vi "LIN UDS Response.vi"(6 "TimeOutMs":i32, 7 "pResData":u8[](array[numeric])=array[4097 elements], 8 "error in (no error)":errorcluster, 9 "pUDSAddr":T1, 10 "LINIndex":u8, 11 "DevHandle":i32) -> (0 "error out":errorcluster, 1 "pUDSAddr out":T1, 3 "function return":i32, 5 "pResData out":u8[](array[numeric]))   [LabVIEW 2010, in "lin_uds.lvlib"]
doc: "int WINAPI LIN_UDS_Response(int DevHandle,unsigned char LINIndex,LIN_UDS_ADDR *pUDSAddr,unsigned char *pResData,int TimeOutMs);"
uses:
  lin_uds.lvlib
  USB2XXX/trunk/USB2XXX/USB2XXX/vs2010/Release/USB2XXX.dll
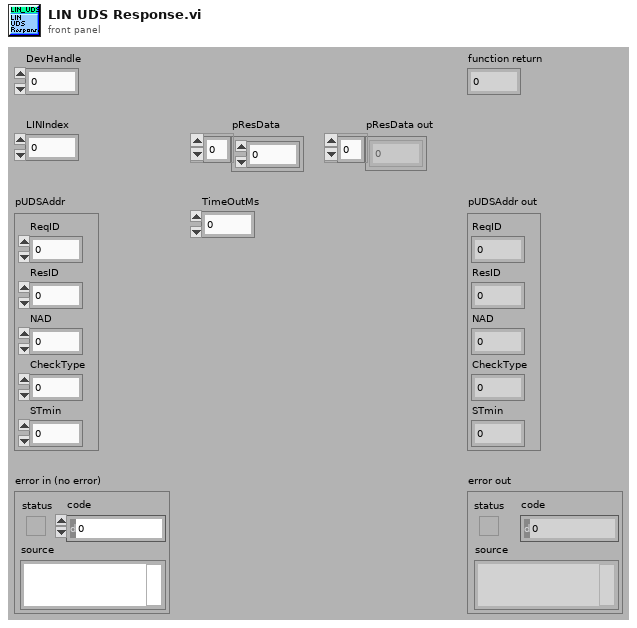
[diagram p1: front panel]
types:
  T1 = cluster{"ReqID":u8, "ResID":u8, "NAD":u8, "CheckType":u8, "STmin":u8}
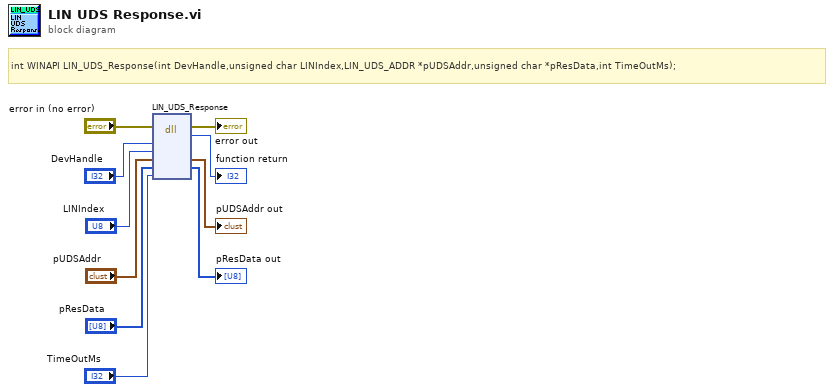
[diagram p0: block diagram]
diagram:
  # "int WINAPI LIN_UDS_Response(int DevHandle,unsigned char LINIndex,LIN_UDS_ADDR *pUDSAddr,unsigned char *pResData,int TimeOutMs);"
  n1 = dll-call lib="E:/OtherWork/STM32/USB2XXX/trunk/USB2XXX/USB2XXX/vs2010/Release/USB2XXX.*" fn="LIN_UDS_Response"(error in="error in (no error)", "DevHandle"="DevHandle", "LINIndex"="LINIndex", "pUDSAddr"="pUDSAddr", "pResData"="pResData", "TimeOutMs"="TimeOutMs") -> (error out=→"error out":errorcluster, →"function return":i32, "pUDSAddr"=→"pUDSAddr out":T1, "pResData"=→"pResData out":u8[])  [unwired: 5 in, 1 out]
